vi "VI dado random.vi"() -> ()   [LabVIEW 2017]
panel:
  in  "stop":bool
  out "4":bool
  out "7":bool
  out "6":bool
  out "5":bool
  out "3":bool
  out "2":bool
  out "1":bool
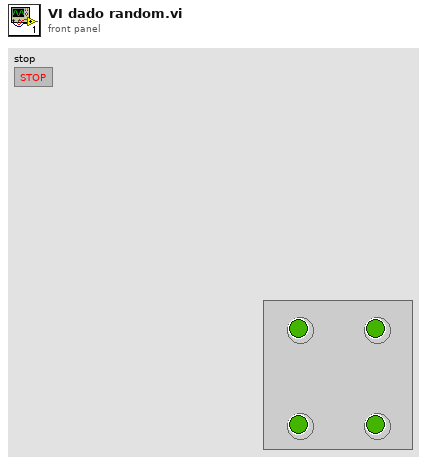
[diagram p1: front panel]
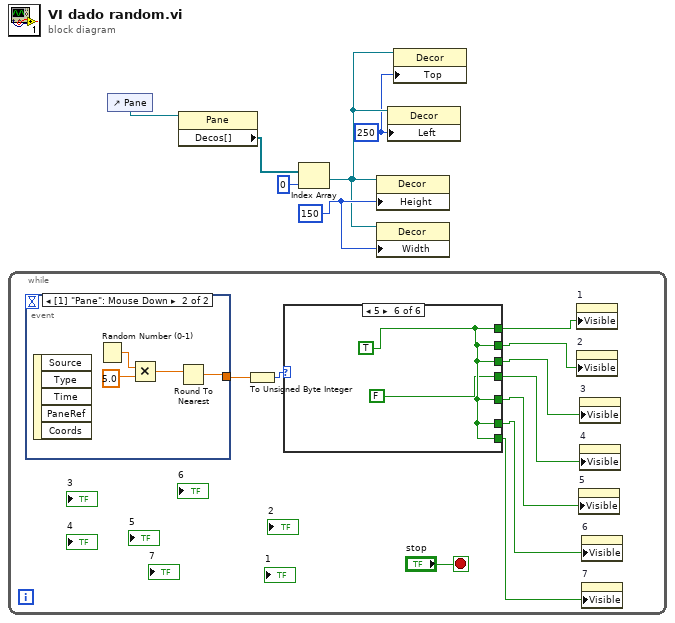
[diagram p0: block diagram]
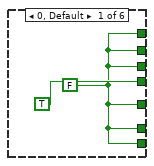
[diagram p2: hidden frame]
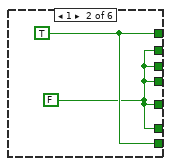
[diagram p3: hidden frame]
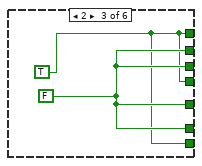
[diagram p4: hidden frame]
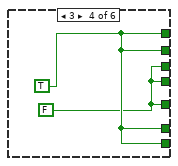
[diagram p5: hidden frame]
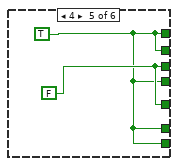
[diagram p6: hidden frame]
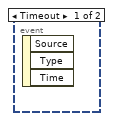
[diagram p7: hidden frame]
diagram:
  w1 = 250 ("Position:Left")
  w3 = 150 ("index")
  n1 = while {
    stop <- "stop" stop-if-true
    n2 = event shown="[1] \"Pane\": Mouse Down" {
      selector: _ -> [_ _]
      dyn-events: _ -> [_ _]
      timeout: _ -> [_ _]
      tunnel: [_ w32] -> w15
      event Timeout {
        n3 = event-data() -> ()  [unwired: 1 in, 3 out]
      }
      event Mouse Down {
        n4 = event-data() -> ()  [unwired: 1 in, 5 out]
        n5 = Random Number (0-1)() -> (number: 0 to 1=w31:dbl)
        n6 = Multiply(x=w31, y=5.0) -> (x*y=w29:dbl)
        n7 = Round To Nearest(number=w29) -> (nearest integer value=w32:dbl)
      }
    }
    n8 = To Unsigned Byte Integer(number=w15) -> (unsigned 8bit integer=w16:u8)
    n9 = case shown="5" w16 {
      tunnel: [w17 w20 w21 w24 w25 w28] -> w13
      tunnel: [w17 w19 w22 w24 w25 w28] -> w12
      tunnel: [w17 w19 w22 w23 w26 w28] -> w11
      tunnel: [TRUE w19 w21 w23 w25 FALSE] -> w10
      tunnel: [w17 w19 w22 w23 w26 w28] -> w9
      tunnel: [w17 w19 w22 w24 w25 w28] -> w8
      tunnel: [w17 w20 w21 w24 w25 w28] -> w7
      frame 0, Default {
        w17 = FALSE
      }
      frame 1 {
        w19 = FALSE
        w20 = TRUE
      }
      frame 2 {
        w22 = FALSE
        w21 = TRUE
      }
      frame 3 {
        w23 = FALSE
        w24 = TRUE
      }
      frame 4 {
        w26 = FALSE
        w25 = TRUE
      }
      frame 5 {
        w28 = TRUE
      }
    }
    n10 = property on="1" class="Bool (strict)"("Visible"=w13) -> ()  [unwired: 2 in, 2 out]
    n11 = property on="2" class="Bool (strict)"("Visible"=w12) -> ()  [unwired: 2 in, 2 out]
    n12 = property on="5" class="Bool (strict)"("Visible"=w9) -> ()  [unwired: 2 in, 2 out]
    n13 = property on="3" class="Bool (strict)"("Visible"=w11) -> ()  [unwired: 2 in, 2 out]
    n14 = property on="4" class="Bool (strict)"("Visible"=w10) -> ()  [unwired: 2 in, 2 out]
    n15 = property on="6" class="Bool (strict)"("Visible"=w8) -> ()  [unwired: 2 in, 2 out]
    n16 = property on="7" class="Bool (strict)"("Visible"=w7) -> ()  [unwired: 2 in, 2 out]
  }
  n17 = control-ref of="Pane"() -> (w6:refnum<vi>)
  n18 = property class="Pane"(reference=w6) -> ("Decos[]"=w5:refnum<vi>[])  [unwired: 1 in, 2 out]
  n19 = Index Array(array=w5, index=0) -> (element=w2:refnum<vi>)
  n20 = property class="Decor"(reference=w2, "Height"=w3) -> ()  [unwired: 1 in, 2 out]
  n21 = property class="Decor"(reference=w2, "Width"=w3) -> ()  [unwired: 1 in, 2 out]
  n22 = property class="Decor"(reference=w2, "Left"=w1) -> ()  [unwired: 1 in, 2 out]
  n23 = property class="Decor"(reference=w2, "Top"=w1) -> ()  [unwired: 1 in, 2 out]
